vi "AlazarReadRegister.vi"(4 "error in (no error)":errorcluster, 5 "Password":u32, 6 "Offset":u32, 7 "Board Handle":u64) -> (0 "error out":errorcluster, 1 "Return Code":u32, 2 "Value Out":u32, 3 "Board Handle Out":u64)   [LabVIEW 2018]
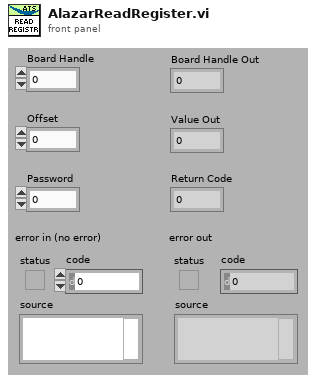
[diagram p1: front panel]
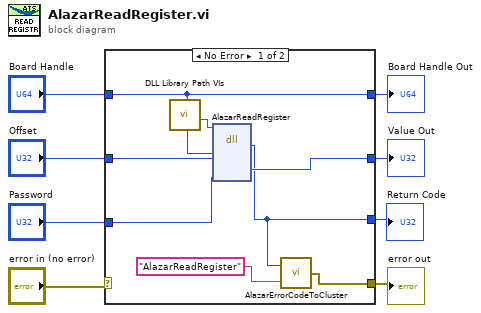
[diagram p0: block diagram]
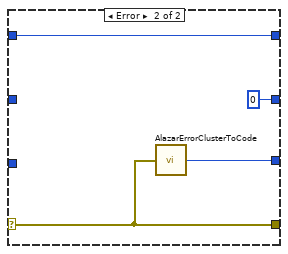
[diagram p2: hidden frame]
diagram:
  n1 = case shown="No Error" "error in (no error)" {
    selector: "error in (no error)" -> [_ w18]
    tunnel: [w10 w18] -> w7
    tunnel: [w13 u32 0] -> w6
    tunnel: [w16 w19] -> w5
    tunnel: "Board Handle" -> [w16 w19]
    tunnel: [w12 w17] -> w3
    tunnel: "Offset" -> [w15 _]
    tunnel: "Password" -> [w14 _]
    frame No Error {
      n2 = call "DLL Library Path VIs.vi"() -> ("Alazar"=w9:path)  [unwired: 9 in, 2 out]
      n3 = dll-call lib="C:/Project/SerialSectOCT - FFT GPU/SerialSectOCT/Labview Software/DLL/ATSApi.dll" fn="AlazarReadRegister"(path in=w9, "handle"=w16, "offset"=w15, "password"=w14) -> ("return type"=w12:u32, "retVal"=w13:u32)  [unwired: 6 in, 2 out]
      n4 = call "AlazarErrorCodeToCluster.vi"("Message"="AlazarReadRegister", "Error Code"=w12) -> ("error out"=w10:errorcluster)
    }
    frame Error {
      n5 = call "AlazarErrorClusterToCode.vi"("error in (no error)"=w18) -> ("Error Code"=w17:u32)
    }
  }
  "Board Handle Out" <- w5
  "Value Out" <- w6
  "error out" <- w7
  "Return Code" <- w3
